vi "loadDailyReport.vi"(10 "error in (no error)":errorcluster) -> (2 "error out":errorcluster)   [LabVIEW 2012]
uses:
  <vilib>/addons/database/Auxilliary.llb/DB Tools Cursor Type.ctl
  <vilib>/addons/database/Connection.llb/DB Tools Open Connec (Path).vi
  <vilib>/addons/database/Connection.llb/Conn Execute.vi
  <vilib>/addons/database/Recordset.llb/Rec Destroy - Connection.vi
  <vilib>/addons/database/NI_Database_API.lvlib
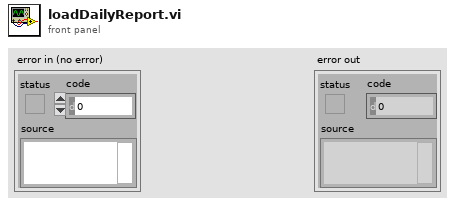
[diagram p1: front panel]
types:
  T1 = typedef "NI_Database_API.lvlib/DB Tools Cursor Type.ctl" = enum16{"forward-only", "keyset", "dynamic", "static"}
  T2 = typedef "NI_Database_API.lvlib/Conn ObjectReference.ctl" = refnum<k1>
  T3 = typedef "NI_Database_API.lvlib/Rec ObjectReference.ctl" = refnum<k1>
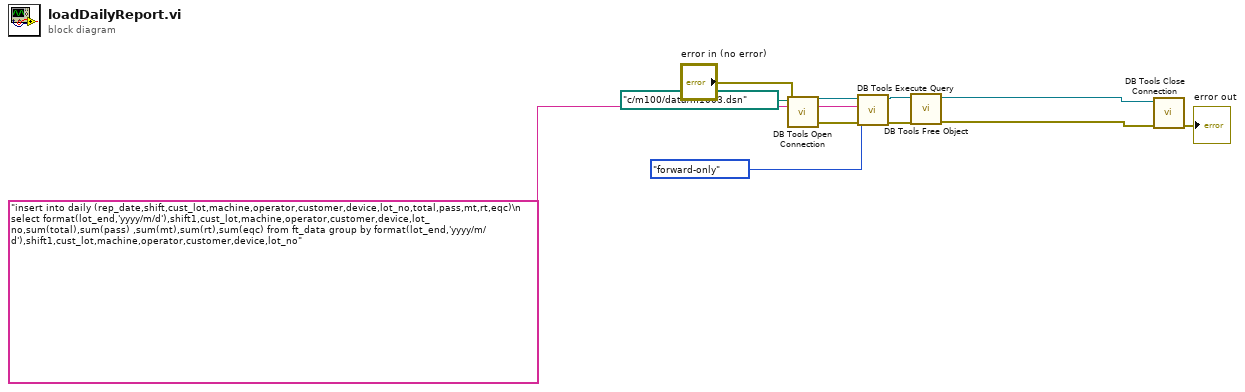
[diagram p0: block diagram]
diagram:
  n1 = call-poly <vilib>:"DB Tools Open Connection.vi"("error in (no error)"="error in (no error)", "connection information"=path "c:/m100/data/m1003.dsn") -> ("error out"=w9:errorcluster, "connection reference"=w10:T2)  [unwired: 6 in]
  n2 = call-poly <vilib>:"DB Tools Execute Query.vi"("error in (no error)"=w9, "cursor type"=DB_Tools_Cursor_Type."forward-only", "SQL query"="insert into daily (rep_date,shift,cust_lot,machine,operator,customer,device,lot_no,total,pass,mt,rt,eqc)\n select format(lot_end,'yyyy/m/d'),shift1,cust_lot,machine,operator,customer,device,lot_no,sum(total),sum(pass) ,sum(mt),sum(rt),sum(eqc) from ft_data group by format(lot_end,'yyyy/m/d'),shift1,cust_lot,machine,operator,customer,device,lot_no", "connection reference"=w10) -> ("error out"=w7:errorcluster, "recordset reference"=w6:T3)  [unwired: 4 in]
  n3 = call-poly <vilib>:"DB Tools Free Object.vi"("error in (no error)"=w7, "recordset reference"=w6) -> ("error out"=w4:errorcluster, "connection reference"=w3:T2)  [unwired: 8 in]
  n4 = call <vilib>:"DB Tools Close Connection.vi"("error in (no error)"=w4, "connection reference"=w3) -> ("error out"=→"error out":errorcluster)  [unwired: 5 in]
